vi "Natural String Comparison.vi"(10 "String 2":string, 11 "String 1":string) -> (3 "String 1 <= String 2":bool)   [LabVIEW 2020, in "UI Common.lvlib"]
uses:
  UI Common.lvlib
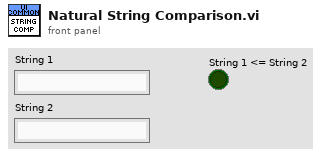
[diagram p1: front panel]
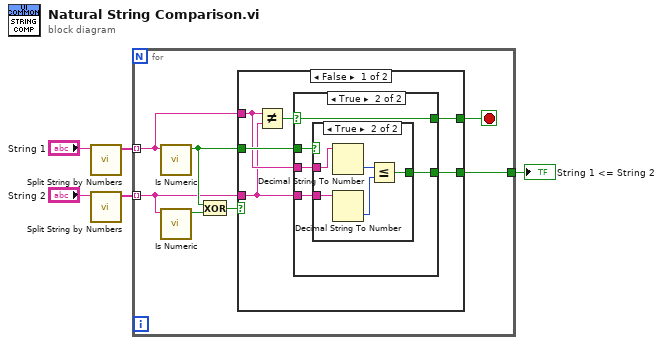
[diagram p0: block diagram]
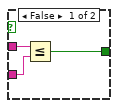
[diagram p3: hidden frame]
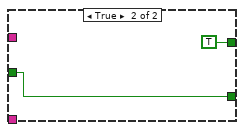
[diagram p4: hidden frame]
diagram:
  n1 = call "Split String by Numbers.vi"("String"="String 1") -> ("Array"=w4:string[])  [unwired: 10 in]
  n2 = call "Split String by Numbers.vi"("String"="String 2") -> ("Array"=w2:string[])  [unwired: 10 in]
  n3 = for {
    tunnel: w4 -> [w7] mode=indexing
    tunnel: w2 -> [w6] mode=indexing
    tunnel: [w9] -> w1
    stop <- w8 stop-if-true
    n4 = call "Is Numeric.vi"("input string"=w7) -> ("is numeric?"=w10:bool)  [unwired: 10 in]
    n5 = call "Is Numeric.vi"("input string"=w6) -> ("is numeric?"=w12:bool)  [unwired: 10 in]
    n6 = Exclusive Or(1:w12, 2:w10) -> (0:w11:bool)
    n7 = case shown="False" w11 {
      tunnel: [w17 w33] -> w9
      tunnel: w10 -> [w18 w33]
      tunnel: [w13 TRUE] -> w8
      tunnel: w7 -> [w16 _]
      tunnel: w6 -> [w15 _]
      frame False {
        n8 = Not Equal?(x=w16, y=w15) -> (x != y?=w14:bool)
        n9 = case shown="True" w14 {
          selector: w14 -> [w19 w20]
          tunnel: w18 -> [_ w24]
          tunnel: [_ w23] -> w17
          tunnel: w16 -> [_ w22]
          tunnel: w15 -> [_ w21]
          tunnel: [w19 w20] -> w13
          frame False {
          }
          frame True {
            n10 = case shown="True" w24 {
              tunnel: w22 -> [w27 w32]
              tunnel: w21 -> [w26 w31]
              tunnel: [w25 w28] -> w23
              frame False {
                n11 = Less Or Equal?(x=w27, y=w26) -> (x <= y?=w25:bool)
              }
              frame True {
                n12 = Decimal String To Number(string=w32) -> (number=w30:i32)  [unwired: 2 in, 1 out]
                n13 = Decimal String To Number(string=w31) -> (number=w29:i32)  [unwired: 2 in, 1 out]
                n14 = Less Or Equal?(x=w30, y=w29) -> (x <= y?=w28:bool)
              }
            }
          }
        }
      }
      frame True {
      }
    }
  }
  "String 1 <= String 2" <- w1
